vi "Bias3_load.vi"() -> ()   [LabVIEW 2025]
panel:
  out "size(s)":i32
  out "Init Data Out":sgl[](array[numeric])
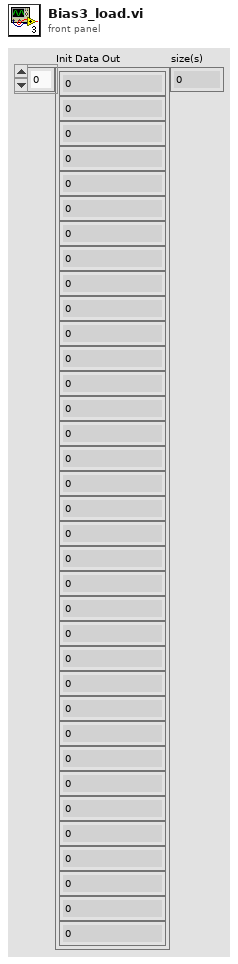
[diagram p1: front panel]
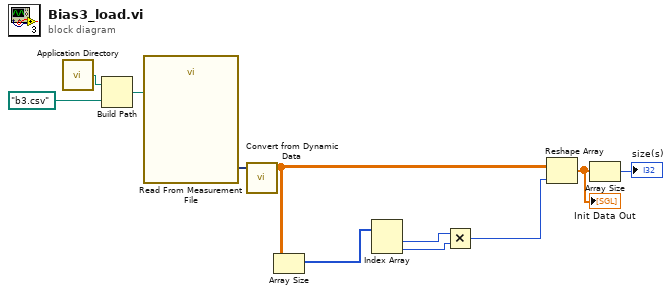
[diagram p0: block diagram]
diagram:
  n1 = call <vilib>:"Application Directory.vi"() -> ("Application Directory"=w10:path)
  n2 = Build Path(base path=w10, name or relative path=path "b3.csv" ("default name")) -> (appended path=w8:path)
  n3 = call "Read From Measurement File"("Filename"=w8) -> ("Signals"=w7:dynamicdata)  [unwired: 5 in, 5 out]
  n4 = call "Convert from Dynamic Data"("Dynamic Data Type"=w7) -> ("Array"=w5:dbl[][])  [unwired: 3 in]
  n5 = Array Size(array=w5) -> (size(s)=w4:i32[])
  n6 = Index Array(array=w4) -> (element #1=w3:i32, element #2=w2:i32)  [unwired: 2 in]
  n7 = Multiply(x=w3, y=w2) -> (x*y=w1:i32)
  n8 = Reshape Array(w5, w1) -> (w6:dbl[])
  "Init Data Out" <- w6
  n9 = Array Size(array=w6) -> (size(s)=→"size(s)":i32)
